vi "Histogram_Manual.vi"(4 "Properties":T1={"Color"=2147483647, "Cumulative"=FALSE, "Normalize"=FALSE, "Line"={"Style"=enum."Automatic", "Color"=2147483647, "Width"=nan}, "Display"={"Alpha"=nan, "Z Order"=nan}} {"Line"."Color" items=["Automatic"=2147483647, "Black"=0, "White"=16777215, "Red"=16711680, "Green"=2263842, "Blue"=255, "Cyan"=65535, "Magenta"=16711935, "Yellow"=16776960]; "Color" items=["Automatic"=2147483647, "Black"=0, "White"=16777215, "Red"=16711680, "Green"=2263842, "Blue"=255, "Cyan"=65535, "Magenta"=16711935, "Yellow"=16776960]}, 6 "Legend Title":string, 7 "Bins":dbl[](array[numeric]), 8 "error in (no error)":errorcluster, 10 "Data":dbl[](array[numeric]), 11 "Plot ID":T6 format="%x") -> (0 "error out":errorcluster, 3 "Plot ID Out":T6 format="%x")   [LabVIEW 2013, in "Advanced Plotting Toolkit.lvlib"]
doc: "Create a 1D bar plot histogram from a data array. Specify the bins explicitly, by providing their edges."
uses:
  Advanced Plotting Toolkit.lvlib
  typedefs/PlotID.ctl
  HistogramProperties.ctl
  typedefs/PlotColor.ctl
  properties/Line.ctl
  properties/Line_Style.ctl
  properties/Display.ctl
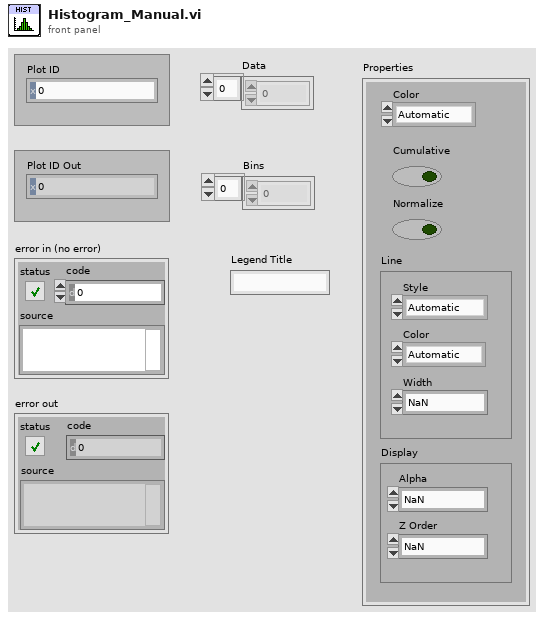
[diagram p1: front panel]
types:
  T1 = typedef "Advanced Plotting Toolkit.lvlib/HistogramProperties.ctl" = cluster{"Color":T2, "Cumulative":bool, "Normalize":bool, "Line":T3, "Display":T5}
  T2 = typedef "Advanced Plotting Toolkit.lvlib/PlotColor.ctl" = u32
  T3 = typedef "Advanced Plotting Toolkit.lvlib/Line.ctl" = cluster{"Style":T4, "Color":T2, "Width":sgl}
  T4 = typedef "Advanced Plotting Toolkit.lvlib/Line_Style.ctl" = enum16{"Automatic", "Solid", "Dashed", "Dotted", "Dash-dot", "Invisible"}
  T5 = typedef "Advanced Plotting Toolkit.lvlib/Display.ctl" = cluster{"Alpha":dbl, "Z Order":dbl}
  T6 = typedef "Advanced Plotting Toolkit.lvlib/PlotID.ctl" = i32
  T7 = typedef "Advanced Plotting Toolkit.lvlib/KeyValue.ctl" = cluster{"Key":string, "Value":string}
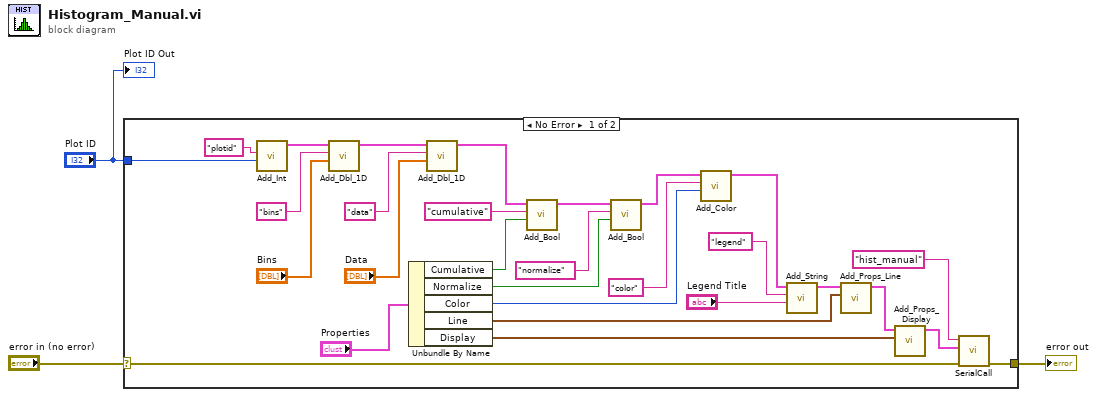
[diagram p0: block diagram]
diagram:
  n1 = case shown="No Error" "error in (no error)" {
    selector: "error in (no error)" -> [w26 w33]
    tunnel: "Plot ID" -> [w32 _]
    tunnel: [w25 w33] -> w1
    frame No Error {
      n2 = call "Add_Int.vi"("Value"=w32, "Key"="plotid") -> ("Keyword Array Out"=w11:T7[])  [unwired: 9 in]
      n3 = call "Add_Dbl_1D.vi"("Value"="Bins", "Key"="bins", "Keyword Array"=w11) -> ("Keyword Array Out"=w10:T7[])  [unwired: 8 in]
      n4 = Unbundle By Name("Properties") -> ("Cumulative"=w22:bool, "Normalize"=w21:bool, "Color"=w19:T2, "Line"=w17:T3, "Display"=w15:T5)
      n5 = call "Add_Dbl_1D.vi"("Value"="Data", "Key"="data", "Keyword Array"=w10) -> ("Keyword Array Out"=w8:T7[])  [unwired: 8 in]
      n6 = call "Add_Bool.vi"("Value"=w22, "Key"="cumulative", "Keyword Array"=w8) -> ("Keyword Array Out"=w20:T7[])  [unwired: 8 in]
      n7 = call "Add_Bool.vi"("Value"=w21, "Key"="normalize", "Keyword Array"=w20) -> ("Keyword Array Out"=w9:T7[])  [unwired: 8 in]
      n8 = call "Add_Color.vi"("Color"=w19, "Key"="color", "Keyword Array"=w9) -> ("Keyword Array Out"=w7:T7[])  [unwired: 8 in]
      n9 = call "Add_String.vi"("Value"="Legend Title", "Key"="legend", "Keyword Array"=w7) -> ("Keyword Array Out"=w6:T7[])  [unwired: 8 in]
      n10 = call "Add_Props_Line.vi"("Line"=w17, "Keyword Array"=w6) -> ("Keyword Array Out"=w16:T7[])  [unwired: 9 in]
      n11 = call "Add_Props_Display.vi"("Display"=w15, "Keyword Array"=w16) -> ("Keyword Array Out"=w14:T7[])  [unwired: 9 in]
      n12 = call "SerialCall.vi"("error in (no error)"=w26, "data"=w14, "Resource"="hist_manual") -> ("error out"=w25:errorcluster)  [unwired: 7 in, 1 out]
    }
    frame Error {
    }
  }
  "error out" <- w1
  "Plot ID Out" <- "Plot ID"
